vi "SeCrTs-Protection Main.vi"() -> ()   [LabVIEW 2022 SP3]
panel:
  out "1 4":bool=TRUE
  out "0 4":bool=TRUE
  out "1 3":bool=TRUE
  out "0 3":bool=TRUE
  in  "Run Ack LOX":bool=TRUE
  in  "Run Ack ATF":bool=TRUE
  out "3":bool=TRUE
  out "2":bool=TRUE
  out "0":bool=TRUE
  out "1":bool=TRUE
  in  "stop":bool
  in  "Under VoltageTBC":dbl=10.0 format="%#_13g"
  in  "Over VoltageTBC":dbl format="%#_13g"
  in  "2 samples- LOX Irms TBC":dbl=400.0 format="%#_13g"
  in  "TBC 10 samples - LOX Irms":dbl=400.0 format="%#_13g"
  in  "Unbalanced TBC - LOX Irms":dbl=400.0 format="%#_13g"
  in  "Unbalanced TBC - ATF Irms":dbl=400.0 format="%#_13g"
  in  "10 samples - ATF Irms TBC":dbl=400.0 format="%#_13g"
  in  "2 samples-ATF Irms TBC":dbl=400.0 format="%#_13g"
  in  "IDC Set Point":dbl format="%#_13g"
  in  "RMS":waveform(dbl)[](array[waveform])=[{"t0"=timestamp(34200 s since 1904-01-01), "dt"=1.0, "Y"=[5.0, 5.0, 5.0, 5.0, 5.0, 5.0, 5.0, 5.0, 5.0, 5.0]}, {"t0"=timestamp(0 s since 1904-01-01), "dt"=1.0, "Y"=[5.0, 5.0, 5.0, 5.0, 5.0, 5.0, 5.0, 5.0, 5.0, 5.0, 4.0, 4.0, 4.0, 4.0, 4.0]}, {"t0"=timestamp(0 s since 1904-01-01), "dt"=1.0, "Y"=[5.0, 5.0, 5.0, 5.0, 5.0, 5.0, 5.0, 5.0, 5.0, 5.0, 5.0, 5.0, 5.0, 5.0, 5.0, 5.0]}, {"t0"=timestamp(0 s since 1904-01-01), "dt"=1.0, "Y"=[5.0, 5.0, 5.0, 5.0, 5.0, 0.0, 5.0, 5.0, 5.0, 5.0, 5.0]}, {"t0"=timestamp(0 s since 1904-01-01), "dt"=1.0, "Y"=[5.0, 5.0, 5.0, 5.0, 5.0, 5.0, 5.0, 5.0, 5.0, 5.0]}, {"t0"=timestamp(0 s since 1904-01-01), "dt"=1.0, "Y"=[5.0, 5.0, 5.0, 5.0, 5.0, 5.0, 5.0, 5.0, 5.0, 5.0]}, {"t0"=timestamp(0 s since 1904-01-01), "dt"=1.0, "Y"=[5.0, 5.0, 5.0, 5.0, 5.0, 5.0, 5.0, 5.0, 5.0, 5.0]}, {"t0"=timestamp(0 s since 1904-01-01), "dt"=1.0, "Y"=[5.0, 5.0, 2.0, 5.0, 5.0, 5.0, 5.0, 5.0, 5.0, 5.0]}, {"t0"=timestamp(0 s since 1904-01-01), "dt"=1.0, "Y"=[5.0, 5.0, 5.0, 5.0, 5.0, 5.0, 5.0, 5.0, 5.0, 5.0]}, {"t0"=timestamp(0 s since 1904-01-01), "dt"=1.0, "Y"=[5.0, 5.0, 5.0, 5.0, 5.0, 5.0, 5.0, 5.0, 5.0, 5.0]}, {"t0"=timestamp(0 s since 1904-01-01), "dt"=1.0, "Y"=[5.0, 5.0, 5.0, 5.0, 5.0, 5.0, 5.0, 5.0, 5.0, 5.0]}]
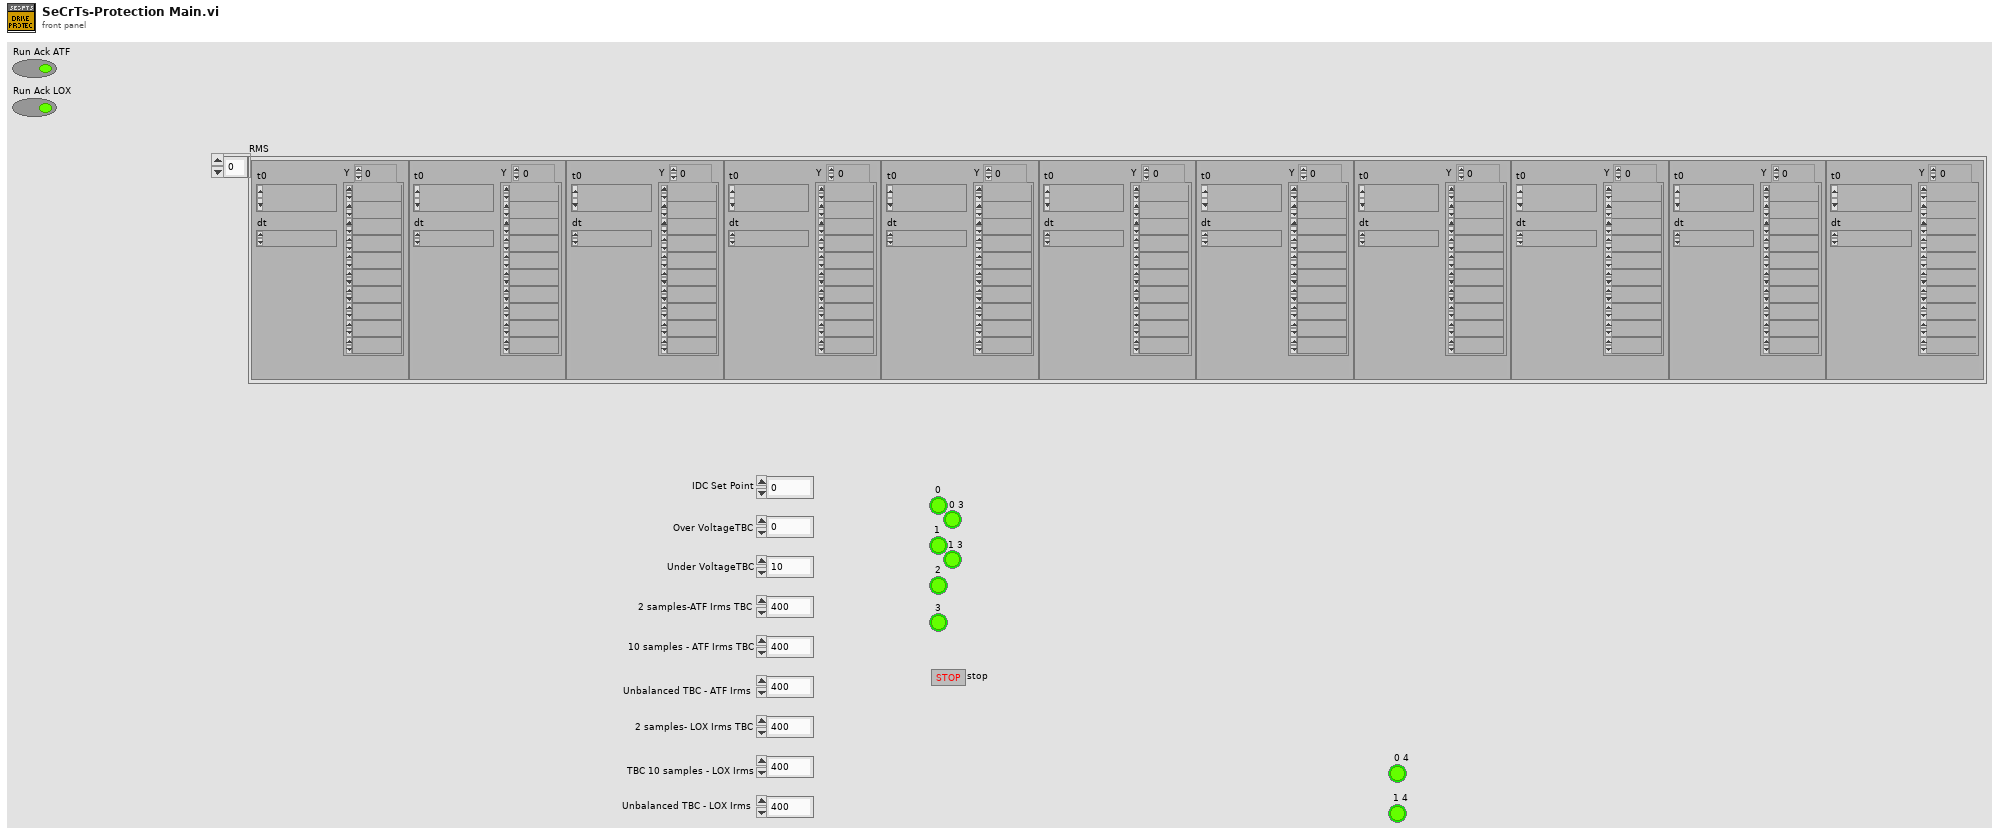
[diagram p1: front panel]
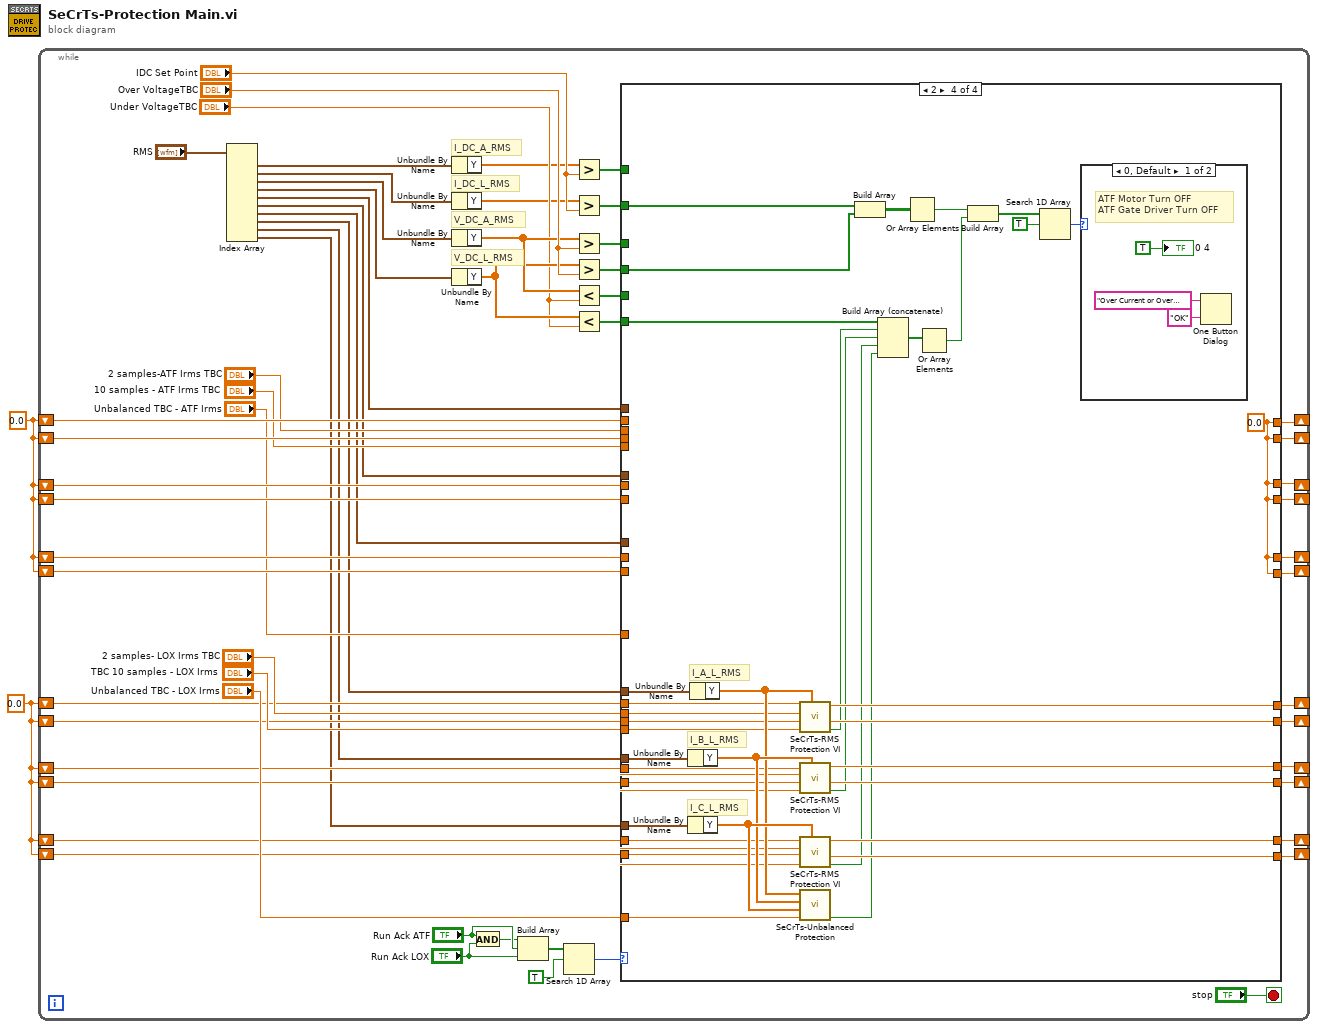
[diagram p0: block diagram]
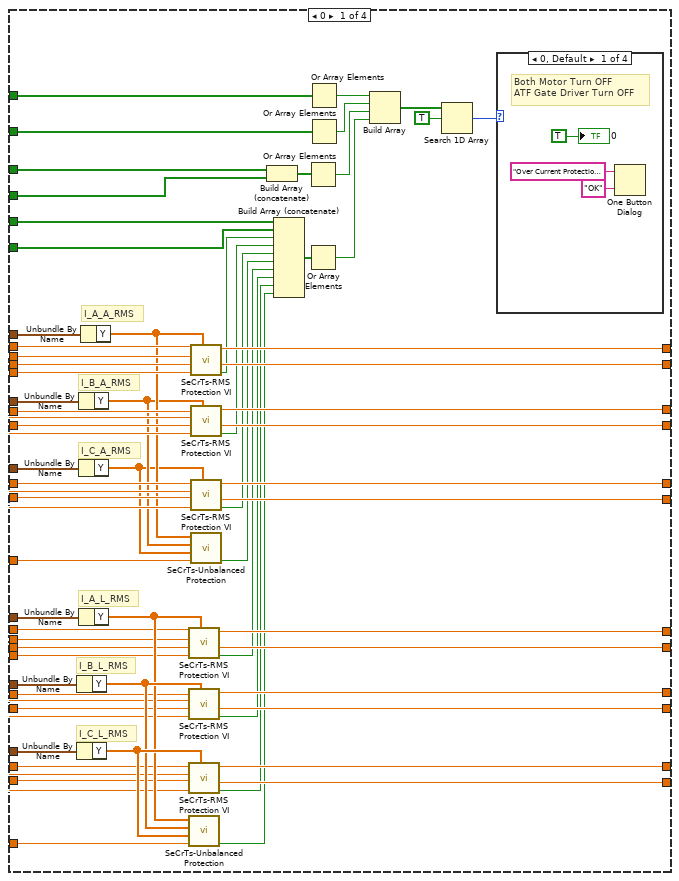
[diagram p2: hidden frame]
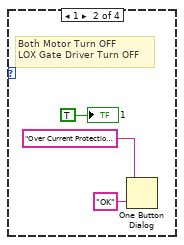
[diagram p3: hidden frame]
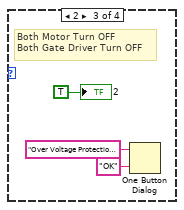
[diagram p4: hidden frame]
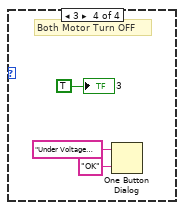
[diagram p5: hidden frame]
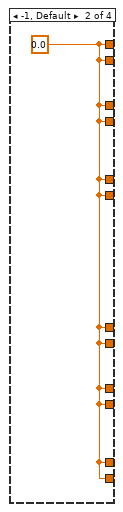
[diagram p6: hidden frame]
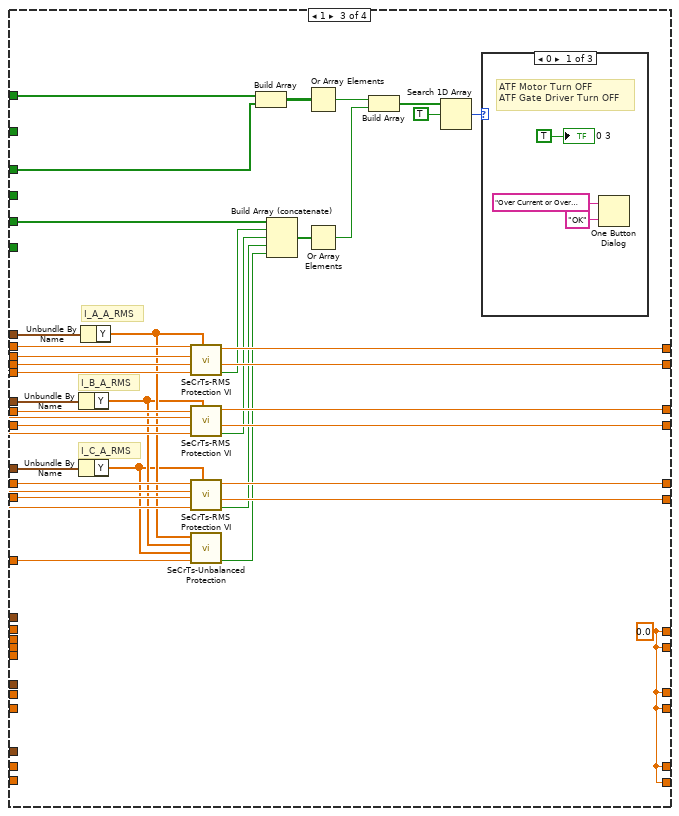
[diagram p7: hidden frame]
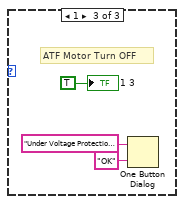
[diagram p9: hidden frame]
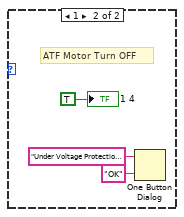
[diagram p10: hidden frame]
diagram:
  w1 = 0.0 ("Trigger 2 times")
  w2 = 0.0 ("Trigger 2 times")
  n1 = while {
    shift-right: [w60] -> _
    shift-left: w2 -> [w61]
    shift-right: [w58] -> _
    shift-left: w2 -> [w59]
    shift-right: [w57] -> _
    shift-left: w2 -> [w50]
    shift-right: [w55] -> _
    shift-left: w2 -> [w56]
    shift-right: [w52] -> _
    shift-left: w2 -> [w54]
    shift-right: [w51] -> _
    shift-left: w2 -> [w53]
    shift-right: [w33] -> _
    shift-left: w1 -> [w32]
    shift-right: [w35] -> _
    shift-left: w1 -> [w34]
    shift-right: [w36] -> _
    shift-left: w1 -> [w43]
    shift-right: [w38] -> _
    shift-left: w1 -> [w37]
    shift-right: [w41] -> _
    shift-left: w1 -> [w39]
    shift-right: [w42] -> _
    shift-left: w1 -> [w40]
    stop <- "stop" stop-if-true
    # "I_DC_L_RMS"
    # "I_DC_A_RMS"
    # "V_DC_L_RMS"
    # "V_DC_A_RMS"
    n2 = Index Array(array="RMS") -> (element #1=w5:waveform(dbl), element #2=w6:waveform(dbl), element #3=w7:waveform(dbl), element #4=w8:waveform(dbl), element #5=w9:waveform(dbl), element #6=w10:waveform(dbl), element #7=w11:waveform(dbl), element #8=w12:waveform(dbl), element #9=w13:waveform(dbl), element #10=w14:waveform(dbl))  [unwired: 10 in]
    n3 = Unbundle By Name(w5) -> ("Y"=w4:dbl[])
    n4 = Unbundle By Name(w6) -> ("Y"=w3:dbl[])
    n5 = Unbundle By Name(w7) -> ("Y"=w30:dbl[])
    n6 = Unbundle By Name(w8) -> ("Y"=w29:dbl[])
    n7 = And(x="Run Ack ATF", y="Run Ack LOX") -> (x .and. y?=w17:bool)
    n8 = Build Array(w17, "Run Ack ATF", "Run Ack LOX") -> (w20:bool[])
    n9 = Search 1D Array(1D array=w20, element=TRUE) -> (index of element=w15:i32)  [unwired: 1 in]
    n10 = Greater?(x=w4, y="IDC Set Point") -> (0:w24:bool[])
    n11 = Greater?(x=w3, y="IDC Set Point") -> (0:w23:bool[])
    n12 = Greater?(x=w30, y="Over VoltageTBC") -> (0:w22:bool[])
    n13 = Greater?(x=w29, y="Over VoltageTBC") -> (0:w21:bool[])
    n14 = Less?(x=w30, y="Under VoltageTBC") -> (x < y?=w28:bool[])
    n15 = Less?(x=w29, y="Under VoltageTBC") -> (x < y?=w27:bool[])
    n16 = case shown="2" w15 {
      tunnel: w9 -> [w128 _ w177 _]
      tunnel: w10 -> [w127 _ w176 _]
      tunnel: w11 -> [w126 _ w175 _]
      tunnel: w61 -> [w125 _ w174 _]
      tunnel: [w124 w141 w173 w193] -> w60
      tunnel: w59 -> [w123 _ w172 _]
      tunnel: [w122 w141 w171 w193] -> w58
      tunnel: [w121 w141 w170 w193] -> w57
      tunnel: w56 -> [w120 _ w169 _]
      tunnel: [w119 w141 w168 w193] -> w55
      tunnel: w54 -> [w118 _ w167 _]
      tunnel: w53 -> [w117 _ w166 _]
      tunnel: [w116 w141 w165 w193] -> w52
      tunnel: [w115 w141 w164 w193] -> w51
      tunnel: w50 -> [w114 _ w163 _]
      tunnel: "2 samples-ATF Irms TBC" -> [w113 _ w162 _]
      tunnel: "10 samples - ATF Irms TBC" -> [w112 _ w161 _]
      tunnel: "Unbalanced TBC - ATF Irms" -> [w108 _ w157 _]
      tunnel: "Unbalanced TBC - LOX Irms" -> [w107 _ _ w219]
      tunnel: "TBC 10 samples - LOX Irms" -> [w103 _ _ w215]
      tunnel: "2 samples- LOX Irms TBC" -> [w102 _ _ w214]
      tunnel: w43 -> [w101 _ _ w213]
      tunnel: [w100 w141 w146 w212] -> w42
      tunnel: [w99 w141 w146 w211] -> w41
      tunnel: w40 -> [w98 _ _ w210]
      tunnel: w39 -> [w97 _ _ w209]
      tunnel: [w96 w141 w146 w208] -> w38
      tunnel: w37 -> [w95 _ _ w207]
      tunnel: [w94 w141 w146 w206] -> w36
      tunnel: [w93 w141 w146 w205] -> w35
      tunnel: w34 -> [w92 _ _ w204]
      tunnel: [w91 w141 w146 w203] -> w33
      tunnel: w32 -> [w90 _ _ w202]
      tunnel: w12 -> [w89 _ _ w201]
      tunnel: w13 -> [w88 _ _ w200]
      tunnel: w14 -> [w87 _ _ w199]
      tunnel: w28 -> [w78 _ w152 _]
      tunnel: w27 -> [w77 _ _ w184]
      tunnel: w24 -> [w73 _ w145 _]
      tunnel: w23 -> [w72 _ _ w188]
      tunnel: w22 -> [w69 _ w144 _]
      tunnel: w21 -> [w68 _ _ w187]
      frame 0 {
        # "I_C_L_RMS"
        # "I_B_L_RMS"
        # "I_A_L_RMS"
        # "I_C_A_RMS"
        # "I_B_A_RMS"
        # "I_A_A_RMS"
        n17 = Unbundle By Name(w88) -> ("Y"=w105:dbl[])
        n18 = Unbundle By Name(w87) -> ("Y"=w106:dbl[])
        n19 = Unbundle By Name(w127) -> ("Y"=w110:dbl[])
        n20 = Unbundle By Name(w126) -> ("Y"=w109:dbl[])
        n21 = Unbundle By Name(w89) -> ("Y"=w104:dbl[])
        n22 = Unbundle By Name(w128) -> ("Y"=w111:dbl[])
        n23 = call "SeCrTs-RMS Protection VI.vi"("RMS Value"=w104, "10 Amps"=w103, "Trigger 10 times"=w92, "5 Amps"=w102, "Trigger 2 times"=w90) -> ("Trigger"=w82:bool, "Trigger 10 out"=w93:dbl, "Trigger 2 out"=w91:dbl)  [unwired: 4 in]
        n24 = call "SeCrTs-RMS Protection VI.vi"("RMS Value"=w105, "10 Amps"=w103, "Trigger 10 times"=w95, "5 Amps"=w102, "Trigger 2 times"=w101) -> ("Trigger"=w81:bool, "Trigger 10 out"=w96:dbl, "Trigger 2 out"=w94:dbl)  [unwired: 4 in]
        n25 = call "SeCrTs-RMS Protection VI.vi"("RMS Value"=w106, "10 Amps"=w103, "Trigger 10 times"=w98, "5 Amps"=w102, "Trigger 2 times"=w97) -> ("Trigger"=w80:bool, "Trigger 10 out"=w100:dbl, "Trigger 2 out"=w99:dbl)  [unwired: 4 in]
        n26 = call "SeCrTs-Unbalanced Protection.vi"("Common Threshold"=w107, "RMS Ic"=w106, "RMS Ib"=w105, "RMS Ia"=w104) -> ("Overall"=w79:bool)  [unwired: 7 in]
        n27 = call "SeCrTs-RMS Protection VI.vi"("RMS Value"=w111, "10 Amps"=w112, "Trigger 10 times"=w123, "5 Amps"=w113, "Trigger 2 times"=w125) -> ("Trigger"=w86:bool, "Trigger 10 out"=w122:dbl, "Trigger 2 out"=w124:dbl)  [unwired: 4 in]
        n28 = call "SeCrTs-RMS Protection VI.vi"("RMS Value"=w110, "10 Amps"=w112, "Trigger 10 times"=w120, "5 Amps"=w113, "Trigger 2 times"=w114) -> ("Trigger"=w85:bool, "Trigger 10 out"=w119:dbl, "Trigger 2 out"=w121:dbl)  [unwired: 4 in]
        n29 = call "SeCrTs-RMS Protection VI.vi"("RMS Value"=w109, "10 Amps"=w112, "Trigger 10 times"=w117, "5 Amps"=w113, "Trigger 2 times"=w118) -> ("Trigger"=w84:bool, "Trigger 10 out"=w115:dbl, "Trigger 2 out"=w116:dbl)  [unwired: 4 in]
        n30 = call "SeCrTs-Unbalanced Protection.vi"("Common Threshold"=w108, "RMS Ic"=w109, "RMS Ib"=w110, "RMS Ia"=w111) -> ("Overall"=w83:bool)  [unwired: 7 in]
        n31 = Build Array (concatenate)(w69, w68) -> (w67:bool[])
        n32 = Build Array (concatenate)(w78, w77, w86, w85, w84, w83, w82, w81, w80, w79) -> (w65:bool[])
        n33 = Or Array Elements(Boolean array=w67) -> (logical OR=w66:bool)
        n34 = Or Array Elements(Boolean array=w65) -> (logical OR=w64:bool)
        n35 = Or Array Elements(Boolean array=w73) -> (logical OR=w71:bool)
        n36 = Or Array Elements(Boolean array=w72) -> (logical OR=w70:bool)
        n37 = Build Array(w71, w70, w66, w64) -> (w75:bool[])
        n38 = Search 1D Array(1D array=w75, element=TRUE ("Overall")) -> (index of element=w74:i32)  [unwired: 1 in]
        n39 = case shown="0, Default" w74 {
          frame 0, Default {
            # "Both Motor Turn OFF\nATF Gate Driver Turn OFF"
            n40 = One Button Dialog(message="Over Current Protection ATF is Trigger", button name ("OK")="OK") -> ()  [unwired: 1 out]
            "0" <- TRUE
          }
          frame 1 {
            # "Both Motor Turn OFF\nLOX Gate Driver Turn OFF"
            n41 = One Button Dialog(message="Over Current Protection LOX is Trigger", button name ("OK")="OK") -> ()  [unwired: 1 out]
            "1" <- TRUE
          }
          frame 2 {
            # "Both Motor Turn OFF\nBoth Gate Driver Turn OFF"
            n42 = One Button Dialog(message="Over Voltage Protection Trigger", button name ("OK")="OK") -> ()  [unwired: 1 out]
            "2" <- TRUE
          }
          frame 3 {
            # "Both Motor Turn OFF"
            n43 = One Button Dialog(message="Under Voltage Protection or Irms is Trigger", button name ("OK")="OK") -> ()  [unwired: 1 out]
            "3" <- TRUE
          }
        }
      }
      frame -1, Default {
        w141 = 0.0 ("Trigger 2 out")
      }
      frame 1 {
        w146 = 0.0 ("Trigger 2 out")
        # "I_C_A_RMS"
        # "I_B_A_RMS"
        # "I_A_A_RMS"
        n44 = Unbundle By Name(w176) -> ("Y"=w159:dbl[])
        n45 = Unbundle By Name(w175) -> ("Y"=w158:dbl[])
        n46 = Unbundle By Name(w177) -> ("Y"=w160:dbl[])
        n47 = call "SeCrTs-RMS Protection VI.vi"("RMS Value"=w160, "10 Amps"=w161, "Trigger 10 times"=w172, "5 Amps"=w162, "Trigger 2 times"=w174) -> ("Trigger"=w156:bool, "Trigger 10 out"=w171:dbl, "Trigger 2 out"=w173:dbl)  [unwired: 4 in]
        n48 = call "SeCrTs-RMS Protection VI.vi"("RMS Value"=w159, "10 Amps"=w161, "Trigger 10 times"=w169, "5 Amps"=w162, "Trigger 2 times"=w163) -> ("Trigger"=w155:bool, "Trigger 10 out"=w168:dbl, "Trigger 2 out"=w170:dbl)  [unwired: 4 in]
        n49 = call "SeCrTs-RMS Protection VI.vi"("RMS Value"=w158, "10 Amps"=w161, "Trigger 10 times"=w166, "5 Amps"=w162, "Trigger 2 times"=w167) -> ("Trigger"=w154:bool, "Trigger 10 out"=w164:dbl, "Trigger 2 out"=w165:dbl)  [unwired: 4 in]
        n50 = call "SeCrTs-Unbalanced Protection.vi"("Common Threshold"=w157, "RMS Ic"=w158, "RMS Ib"=w159, "RMS Ia"=w160) -> ("Overall"=w153:bool)  [unwired: 7 in]
        n51 = Build Array(w145, w144) -> (w143:bool[][])
        n52 = Build Array (concatenate)(w152, w156, w155, w154, w153) -> (w147:bool[])
        n53 = Or Array Elements(Boolean array=w143) -> (logical OR=w148:bool)
        n54 = Or Array Elements(Boolean array=w147) -> (logical OR=w142:bool)
        n55 = Build Array(w148, w142) -> (w150:bool[])
        n56 = Search 1D Array(1D array=w150, element=TRUE ("Overall")) -> (index of element=w149:i32)  [unwired: 1 in]
        n57 = case shown="0" w149 {
          frame 0 {
            # "ATF Motor Turn OFF\nATF Gate Driver Turn OFF"
            n58 = One Button Dialog(message="Over Current or Over VOltage Protection is Triggered", button name ("OK")="OK") -> ()  [unwired: 1 out]
            "0 3" <- TRUE
          }
          frame -1, Default {
          }
          frame 1 {
            # "ATF Motor Turn OFF"
            n59 = One Button Dialog(message="Under Voltage Protection or Irms is Trigger", button name ("OK")="OK") -> ()  [unwired: 1 out]
            "1 3" <- TRUE
          }
        }
      }
      frame 2 {
        w193 = 0.0 ("Trigger 2 out")
        # "I_C_L_RMS"
        # "I_B_L_RMS"
        # "I_A_L_RMS"
        n60 = Unbundle By Name(w200) -> ("Y"=w217:dbl[])
        n61 = Unbundle By Name(w199) -> ("Y"=w218:dbl[])
        n62 = Unbundle By Name(w201) -> ("Y"=w216:dbl[])
        n63 = call "SeCrTs-RMS Protection VI.vi"("RMS Value"=w216, "10 Amps"=w215, "Trigger 10 times"=w204, "5 Amps"=w214, "Trigger 2 times"=w202) -> ("Trigger"=w197:bool, "Trigger 10 out"=w205:dbl, "Trigger 2 out"=w203:dbl)  [unwired: 4 in]
        n64 = call "SeCrTs-RMS Protection VI.vi"("RMS Value"=w217, "10 Amps"=w215, "Trigger 10 times"=w207, "5 Amps"=w214, "Trigger 2 times"=w213) -> ("Trigger"=w196:bool, "Trigger 10 out"=w208:dbl, "Trigger 2 out"=w206:dbl)  [unwired: 4 in]
        n65 = call "SeCrTs-RMS Protection VI.vi"("RMS Value"=w218, "10 Amps"=w215, "Trigger 10 times"=w210, "5 Amps"=w214, "Trigger 2 times"=w209) -> ("Trigger"=w195:bool, "Trigger 10 out"=w212:dbl, "Trigger 2 out"=w211:dbl)  [unwired: 4 in]
        n66 = call "SeCrTs-Unbalanced Protection.vi"("Common Threshold"=w219, "RMS Ic"=w218, "RMS Ib"=w217, "RMS Ia"=w216) -> ("Overall"=w194:bool)  [unwired: 7 in]
        n67 = Build Array(w188, w187) -> (w186:bool[][])
        n68 = Build Array (concatenate)(w184, w197, w196, w195, w194) -> (w198:bool[])
        n69 = Or Array Elements(Boolean array=w186) -> (logical OR=w190:bool)
        n70 = Or Array Elements(Boolean array=w198) -> (logical OR=w185:bool)
        n71 = Build Array(w190, w185) -> (w192:bool[])
        n72 = Search 1D Array(1D array=w192, element=TRUE ("Overall")) -> (index of element=w191:i32)  [unwired: 1 in]
        n73 = case shown="0, Default" w191 {
          frame 0, Default {
            # "ATF Motor Turn OFF\nATF Gate Driver Turn OFF"
            n74 = One Button Dialog(message="Over Current or Over VOltage Protection is Triggered", button name ("OK")="OK") -> ()  [unwired: 1 out]
            "0 4" <- TRUE
          }
          frame 1 {
            # "ATF Motor Turn OFF"
            n75 = One Button Dialog(message="Under Voltage Protection or Irms is Trigger", button name ("OK")="OK") -> ()  [unwired: 1 out]
            "1 4" <- TRUE
          }
        }
      }
    }
  }
